vi "ARP-Create.vi"(1 "Target":cluster{"THA":u8[], "TPA":u8[]}={"THA"=[0, 35, 38, 182, 175, 53], "TPA"=[192, 168, 1, 200]} {"THA" format="%02x"}, 2 "Sender":cluster{"SHA":u8[], "SPA":u8[]}={"SHA"=[0, 80, 67, 160, 161, 162], "SPA"=[192, 168, 1, 201]} {"SHA" format="%02x"}, 3 "Header":T1={"HTYPE"=1, "PTYPE"=2048, "HLEN"=6, "PLEN"=4, "OPER"=2}) -> (0 "Arp Packet (out)":u8[](array[numeric])=[0, 1, 8, 0, 6, 4, 0, 2, 0, 80, 67, 192, 168, 1, 201, 0, 35, 38, 182, 175, 53, 192, 168, 1, 200] format="%02x")   [LabVIEW 2018]
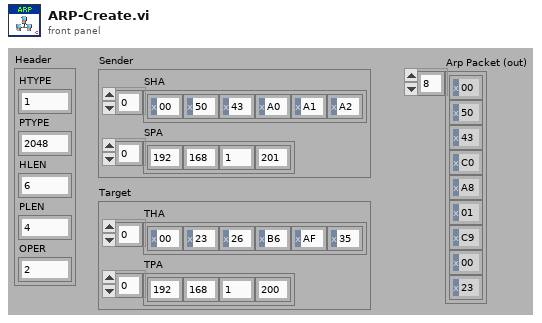
[diagram p1: front panel]
types:
  T1 = cluster{"HTYPE":u16, "PTYPE":u16, "HLEN":u8, "PLEN":u8, "OPER":u16}
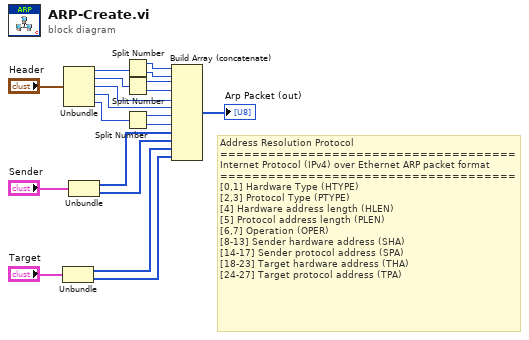
[diagram p0: block diagram]
diagram:
  # "Address Resolution Protocol\n=====================================\nInternet Protocol (IPv4) over Ethernet ARP packet format\n===================================== \n[0,1] Hardware Type (HTYPE)\n[2,3] Protocol Type (PTYPE)\n[4] Hardware address length (HLEN)\n[5] Protocol address length (PLEN)\n[6,7] Operation (OPER)\n[8-13] Sender hardware address (SHA)\n[14-17] Sender protocol address (SPA)\n[18-23] Target hardware address (THA)\n[24-27] Target protocol address (TPA)"
  n1 = Unbundle("Target") -> ("THA"=w18:u8[], "TPA"=w19:u8[])
  n2 = Unbundle("Header") -> ("HTYPE"=w2:u16, "PTYPE"=w3:u16, "HLEN"=w8:u8, "PLEN"=w9:u8, "OPER"=w10:u16)
  n3 = Unbundle("Sender") -> ("SHA"=w16:u8[], "SPA"=w17:u8[])
  n4 = Split Number(x=w2) -> (hi(x)=w4:u8, lo(x)=w5:u8)
  n5 = Split Number(x=w3) -> (hi(x)=w6:u8, lo(x)=w7:u8)
  n6 = Split Number(x=w10) -> (hi(x)=w11:u8, lo(x)=w12:u8)
  n7 = Build Array (concatenate)(w4, w5, w6, w7, w8, w9, w11, w12, w16, w17, w18, w19) -> (→"Arp Packet (out)":u8[])
